vi "RP Active.vi"   [LabVIEW 2025]
doc: "Sets User1 LED on cRIO chassis to illuminated if at least one Remote Panel connection is active to a VI running on the cRIO."
uses:
  <vilib>/NI_Real-Time Target Support.lvlib
types:
  T1 = typedef "LVRemotePanelConnectionsTypeDef.ctl" = cluster{"VI Name":string, "Remote":string, "UserName":string, "Port":i32, "Status":enum32{"Viewing", "Waiting For Control", "Controlling"}, "Create Time":timestamp, "Status Time":timestamp, "Control End Time":timestamp}[]
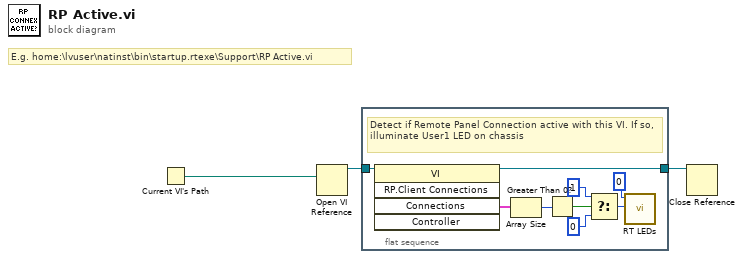
[diagram p0: block diagram]
diagram:
  # "E.g. home:\\lvuser\\natinst\\bin\\startup.rtexe\\Support\\RP Active.vi"
  n1 = Current VI's Path() -> (path=w1:path)
  n2 = Open VI Reference(vi path=w1) -> (vi reference=w3:refnum<vi>)  [unwired: 5 in, 1 out]
  n3 = flat-sequence {
    tunnel: w3 -> [w12]
    tunnel: [w11] -> w2
    frame #0 {
      # "Detect if Remote Panel Connection active with this VI. If so, illuminate User1 LED on chassis"
      n4 = invoke class="VI" method="RP.Client Connections"(reference=w12) -> (reference out=w11:refnum<vi>, "Connections"=w10:T1)  [unwired: 4 in, 3 out]
      n5 = Array Size(array=w10) -> (size(s)=w9:i32)
      n6 = Greater Than 0?(x=w9) -> (x > 0?=w5:bool)
      n7 = Select(t=1 ("State"), s=w5, f=0 ("State")) -> (s? t:f=w4:i32)
      n8 = call <vilib>:"RT LEDs.vi"("State"=w4, "LED Num"=0) -> ()  [unwired: 4 in, 2 out]
    }
  }
  n9 = Close Reference(reference=w2) -> ()  [unwired: 1 in, 1 out]
